vi "UT_get section vim.vi"   [LabVIEW 2020]
uses:
  lib/TOML.lvlib
  <vilib>/addons/_JKI Toolkits/Caraya/classes/Test/Test.lvclass
  <vilib>/addons/_JKI Toolkits/Caraya/classes/Assert/Assert.lvclass
  <vilib>/addons/_JKI Toolkits/Caraya/classes/Assert/Assert Equal Value and Type_Variant.vi
  <vilib>/addons/_JKI Toolkits/Caraya/classes/Assert/Assert Not Error.vi
  <vilib>/addons/_JKI Toolkits/Caraya/classes/Assert/Assert Error.vi
  6f95a99f-c5fd-488e-b143-13ca014596ae.vi
  fe2005f7-26cf-4ff5-b812-afcc3cf71471.vi
  2f48c145-f647-46dc-8eae-f5e8f0a9a1e2.vi
  52f0a0c0-a733-488e-b438-e27a088fc746.vi
  d21704fd-f14a-4858-bc63-1182cd6ab1ef.vi
  14822d35-f4e9-4b7d-b4cf-a580779f7ff3.vi
types:
  T1 = cluster{"string1":string, "string2":string, "string3":string}
  T2 = typedef "TOML.lvlib/TOML Value.ctl" = cluster{"type":enum16{"Table", "Array", "String", "Integer", "Float", "Boolean", "Offset Date-Time", "Local Date-Time", "Local Date", "Local Time", "Path"}, "value":variant}
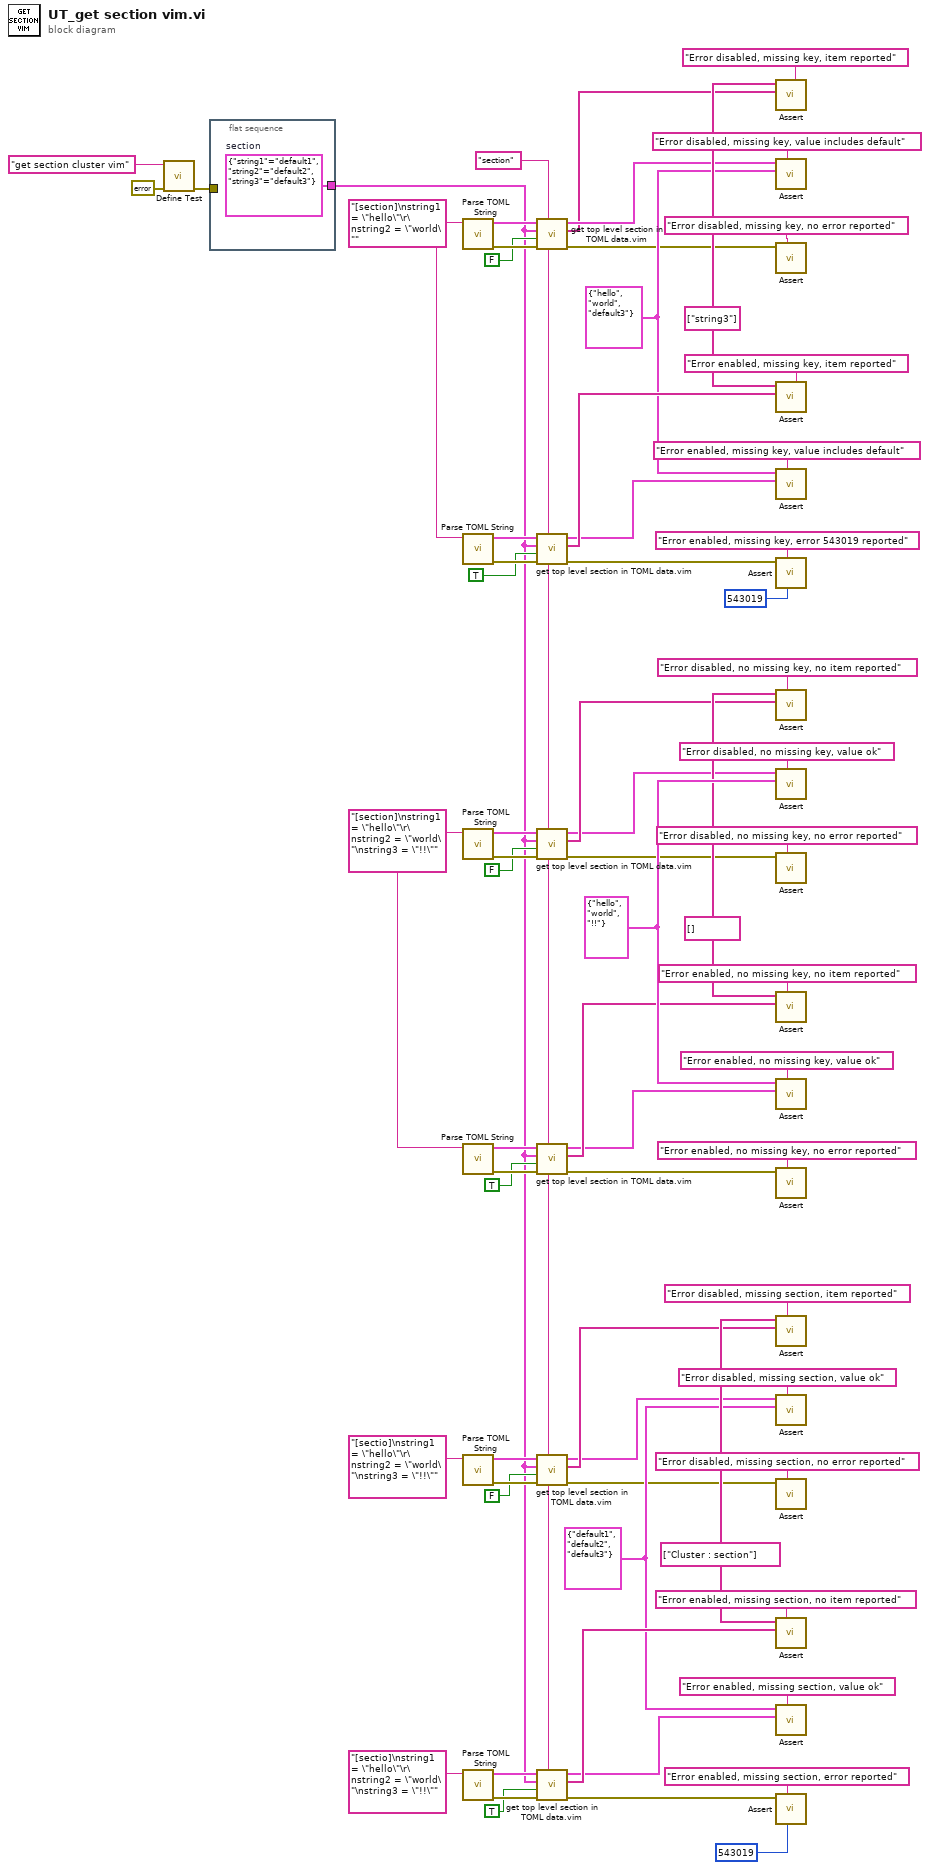
[diagram p0: block diagram]
diagram:
  w3 = "section" ("Section name")
  w23 = T1 {"string1"="default1", "string2"="default2", "string3"="default3"} ("data")
  w30 = string[] ["Cluster : section"] ("Missing elements")
  w49 = T1 {"string1"="hello", "string2"="world", "string3"="!!"} ("data")
  w45 = string[] [] ("Missing elements")
  w50 = T1 {"string1"="hello", "string2"="world", "string3"="default3"} ("data")
  w54 = string[] ["string3"] ("Missing elements")
  w64 = "[section]\nstring1 = \"hello\"\r\nstring2 = \"world\"\nstring3 = \"!!\"" ("x")
  w66 = "[section]\nstring1 = \"hello\"\r\nstring2 = \"world\"" ("x")
  n1 = call <vilib>:"Define Test.vi"("error in (no error)"=errorcluster {"status"=FALSE, "code"=0, "source"=""}, "Label (VI Title)"="get section cluster vim") -> ("error out"=w61:errorcluster)  [unwired: 8 in, 1 out]
  n2 = flat-sequence {
    tunnel: [w72] -> w1
    tunnel: w61 -> [_]
    frame #0 {
      w72 = T1 {"string1"="default1", "string2"="default2", "string3"="default3"}  # section
    }
  }
  n3 = call "Parse TOML String.vi"("String"=w66) -> ("error out"=w71:errorcluster, "Value"=w10:T2)  [unwired: 9 in]
  n4 = call "Parse TOML String.vi"("String"=w66) -> ("error out"=w68:errorcluster, "Value"=w67:T2)  [unwired: 9 in]
  n5 = call "Parse TOML String.vi"("String"=w64) -> ("error out"=w70:errorcluster, "Value"=w69:T2)  [unwired: 9 in]
  n6 = call "Parse TOML String.vi"("String"=w64) -> ("error out"=w65:errorcluster, "Value"=w17:T2)  [unwired: 9 in]
  n7 = call "Parse TOML String.vi"("String"="[sectio]\nstring1 = \"hello\"\r\nstring2 = \"world\"\nstring3 = \"!!\"" ("x")) -> ("error out"=w37:errorcluster, "Value"=w20:T2)  [unwired: 9 in]
  n8 = call "Parse TOML String.vi"("String"="[sectio]\nstring1 = \"hello\"\r\nstring2 = \"world\"\nstring3 = \"!!\"" ("x")) -> ("error out"=w36:errorcluster, "Value"=w35:T2)  [unwired: 9 in]
  n9 = call "get top level section in TOML data.vim"("Section name"=w3, "error in (no error)"=w71, "Error if missing element"=FALSE, "Section datatype"=w1, "Value in"=w10) -> ("error out"=w11:errorcluster, "Missing elements"=w8:string[], "LV Value"=w12:T1)  [unwired: 4 in]
  n10 = call "get top level section in TOML data.vim"("Section name"=w3, "error in (no error)"=w68, "Error if missing element"=TRUE, "Section datatype"=w1, "Value in"=w67) -> ("error out"=w56:errorcluster, "Missing elements"=w58:string[], "LV Value"=w13:T1)  [unwired: 4 in]
  n11 = call "get top level section in TOML data.vim"("Section name"=w3, "error in (no error)"=w70, "Error if missing element"=FALSE, "Section datatype"=w1, "Value in"=w69) -> ("error out"=w14:errorcluster, "Missing elements"=w39:string[], "LV Value"=w15:T1)  [unwired: 4 in]
  n12 = call "get top level section in TOML data.vim"("Section name"=w3, "error in (no error)"=w65, "Error if missing element"=TRUE, "Section datatype"=w1, "Value in"=w17) -> ("error out"=w41:errorcluster, "Missing elements"=w40:string[], "LV Value"=w16:T1)  [unwired: 4 in]
  n13 = call "get top level section in TOML data.vim"("Section name"=w3, "error in (no error)"=w37, "Error if missing element"=FALSE, "Section datatype"=w1, "Value in"=w20) -> ("error out"=w19:errorcluster, "Missing elements"=w24:string[], "LV Value"=w18:T1)  [unwired: 4 in]
  n14 = call "get top level section in TOML data.vim"("Section name"=w3, "error in (no error)"=w36, "Error if missing element"=TRUE, "Section datatype"=w1, "Value in"=w35) -> ("error out"=w26:errorcluster, "Missing elements"=w25:string[], "LV Value"=w21:T1)  [unwired: 4 in]
  n15 = call-poly <vilib>:"Assert.vi"("Label"="Error disabled, missing key, item reported" ("Label (VI Title)"), "Y"=w8, "X"=w54) -> ()  [unwired: 7 in, 2 out]
  n16 = call-poly <vilib>:"Assert.vi"("Label"="Error disabled, missing key, value includes default" ("Label (VI Title)"), "Y"=w50, "X"=w12) -> ()  [unwired: 7 in, 2 out]
  n17 = call-poly <vilib>:"Assert.vi"("Label"="Error disabled, missing key, no error reported" ("Label (VI Title)"), "Not Error?"=w11) -> ()  [unwired: 8 in, 2 out]
  n18 = call-poly <vilib>:"Assert.vi"("Label"="Error enabled, missing key, item reported" ("Label (VI Title)"), "Y"=w58, "X"=w54) -> ()  [unwired: 7 in, 2 out]
  n19 = call-poly <vilib>:"Assert.vi"("Label"="Error enabled, missing key, value includes default" ("Label (VI Title)"), "Y"=w13, "X"=w50) -> ()  [unwired: 7 in, 2 out]
  n20 = call-poly <vilib>:"Assert.vi"("error code (1)"=543019, "Label"="Error enabled, missing key, error 543019 reported" ("Label (VI Title)"), "Error?"=w56) -> ()  [unwired: 7 in, 2 out]
  n21 = call-poly <vilib>:"Assert.vi"("Label"="Error disabled, no missing key, no item reported" ("Label (VI Title)"), "Y"=w39, "X"=w45) -> ()  [unwired: 7 in, 2 out]
  n22 = call-poly <vilib>:"Assert.vi"("Label"="Error disabled, no missing key, value ok" ("Label (VI Title)"), "Y"=w49, "X"=w15) -> ()  [unwired: 7 in, 2 out]
  n23 = call-poly <vilib>:"Assert.vi"("Label"="Error disabled, no missing key, no error reported" ("Label (VI Title)"), "Not Error?"=w14) -> ()  [unwired: 8 in, 2 out]
  n24 = call-poly <vilib>:"Assert.vi"("Label"="Error enabled, no missing key, no item reported" ("Label (VI Title)"), "Y"=w40, "X"=w45) -> ()  [unwired: 7 in, 2 out]
  n25 = call-poly <vilib>:"Assert.vi"("Label"="Error enabled, no missing key, value ok" ("Label (VI Title)"), "Y"=w16, "X"=w49) -> ()  [unwired: 7 in, 2 out]
  n26 = call-poly <vilib>:"Assert.vi"("Label"="Error enabled, no missing key, no error reported" ("Label (VI Title)"), "Not Error?"=w41) -> ()  [unwired: 8 in, 2 out]
  n27 = call-poly <vilib>:"Assert.vi"("Label"="Error disabled, missing section, item reported" ("Label (VI Title)"), "Y"=w24, "X"=w30) -> ()  [unwired: 7 in, 2 out]
  n28 = call-poly <vilib>:"Assert.vi"("Label"="Error disabled, missing section, value ok" ("Label (VI Title)"), "Y"=w23, "X"=w18) -> ()  [unwired: 7 in, 2 out]
  n29 = call-poly <vilib>:"Assert.vi"("Label"="Error disabled, missing section, no error reported" ("Label (VI Title)"), "Not Error?"=w19) -> ()  [unwired: 8 in, 2 out]
  n30 = call-poly <vilib>:"Assert.vi"("Label"="Error enabled, missing section, no item reported" ("Label (VI Title)"), "Y"=w25, "X"=w30) -> ()  [unwired: 7 in, 2 out]
  n31 = call-poly <vilib>:"Assert.vi"("Label"="Error enabled, missing section, value ok" ("Label (VI Title)"), "Y"=w21, "X"=w23) -> ()  [unwired: 7 in, 2 out]
  n32 = call-poly <vilib>:"Assert.vi"("error code (1)"=543019, "Label"="Error enabled, missing section, error reported" ("Label (VI Title)"), "Error?"=w26) -> ()  [unwired: 7 in, 2 out]
